vi "AlliGator Load Calibration Phasor Map.vi"(8 "Error In":errorcluster, 10 "File Path (empty: dialog)":path=path "", 11 "Calibration Phasor Map in":T1={"Phasor Frequency"=80000000.0, "Calibration Lifetime"=1e-09, "ROI Centers"=[], "ROI Descriptors"=[], "Map Resolution X"=0, "Map Resolution Y"=0, "z Array"=[]} {"ROI Descriptors"."Contours"."Type" items=["No Selection", "Point", "Line", "Rectangle", "Oval", "Polygon", "Freehand Region", "Annulus", "Unused2", "Unused3", "Broken Line", "Freehand Line", "Rotated Rectangle"]}) -> (0 "error out":errorcluster, 1 "Phasor Frequency":dbl[unit], 2 "File Path":path, 3 "Calibration Phasor Map out":T1={"Phasor Frequency"=80000000.0, "Calibration Lifetime"=1e-09, "ROI Centers"=[], "ROI Descriptors"=[], "Map Resolution X"=0, "Map Resolution Y"=0, "z Array"=[]} {"ROI Descriptors"."Contours"."Type" items=["No Selection", "Point", "Line", "Rectangle", "Oval", "Polygon", "Freehand Region", "Annulus", "Unused2", "Unused3", "Broken Line", "Freehand Line", "Rotated Rectangle"]}, 4 "Message":string)   [LabVIEW 2021, in "AlliGator Phasor Calibration.lvlib"]
doc: "Loads a <B>Phasor Calibraton Map</B>."
uses:
  AlliGator Phasor Calibration.lvlib
  Phasor/Phasor Calibration Map v2.ctl
  AlliGator Phasor Calibration Map v1.ctl
  c0370fcd-593d-4089-81d1-2cd858bd6d0b.vi
  f35317ec-b920-4f06-9f91-dc9fc3beab4a.vi
  f35317ec-b920-4f06-9f91-dc9fc3beab4a.vi/8a80743f-1319-44c8-96b0-3ef8fc688731.vi
  f35317ec-b920-4f06-9f91-dc9fc3beab4a.vi/931f4f8f-d8c6-4056-833f-5c8fe97b24b9.vi
  <vilib>/JDP Science/JSONtext/JSON text to Variant.vi
  <vilib>/Utility/error.llb/Error Cluster From Error Code.vi
  <vilib>/JDP Science/JSONtext/LVClass Serializer/JSONtext LVClass Serializer.lvclass
  <vilib>/ErrorRing/Error Ring.xnode
  Settings/AlliGator Settings.lvlib
  Time/Time.lvlib
  Phasor/Phasor.lvlib
panel:
  # "see the AlliGator License on the block diagram (Ctrl+E or Window:Show Block Diagram)"
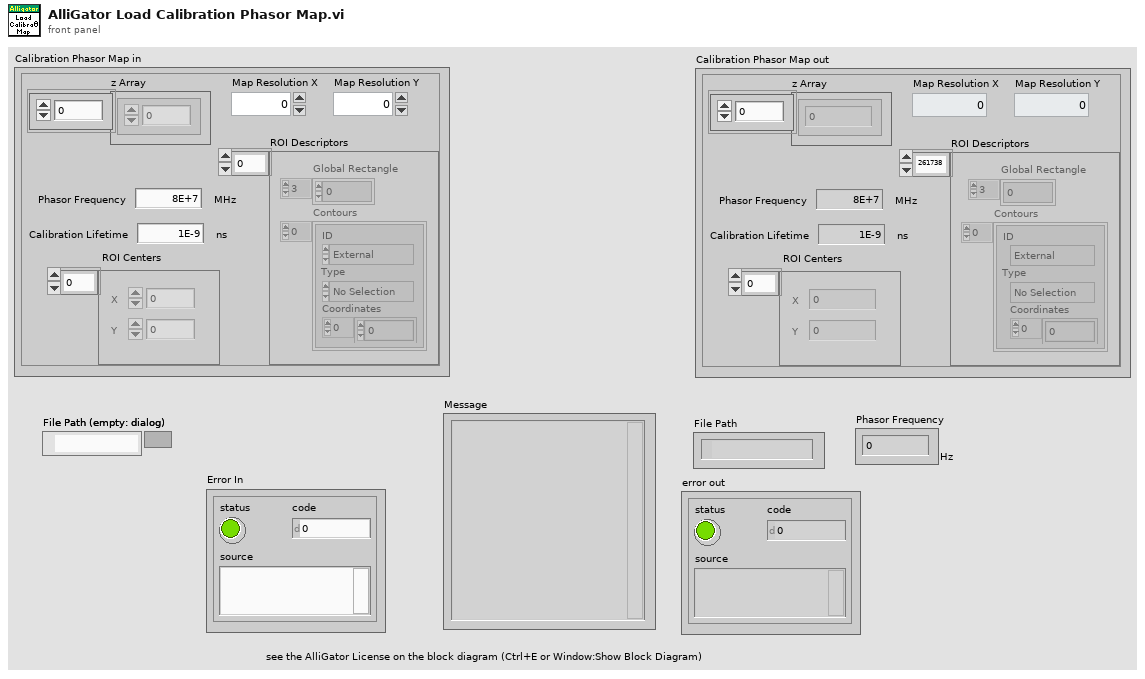
[diagram p1: front panel]
types:
  T1 = typedef "Phasor.lvlib/Phasor Calibration Map v2.ctl" = cluster{"Phasor Frequency":dbl[unit], "Calibration Lifetime":dbl[unit], "ROI Centers":cluster{"X":i32, "Y":i32}[], "ROI Descriptors":T2[], "Map Resolution X":i32, "Map Resolution Y":i32, "z Array":cdb[]}
  T2 = typedef "ROI Descriptor" = cluster{"Global Rectangle":i32[], "Contours":cluster{"ID":enum32{"External", "Internal"}, "Type":u32, "Coordinates":i32[]}[]}
  T3 = typedef "AlliGator Phasor Calibration.lvlib/AlliGator Phasor Calibration Map v1.ctl" = cluster{"m Array":dbl[], "phi Array":dbl[], "Phasor Frequency":dbl[unit], "Calibration Lifetime":dbl[unit], "ROI Centers":cluster{"X":i32, "Y":i32}[], "ROI Descriptors":T2[], "Map Resolution X":i32, "Map Resolution Y":i32}
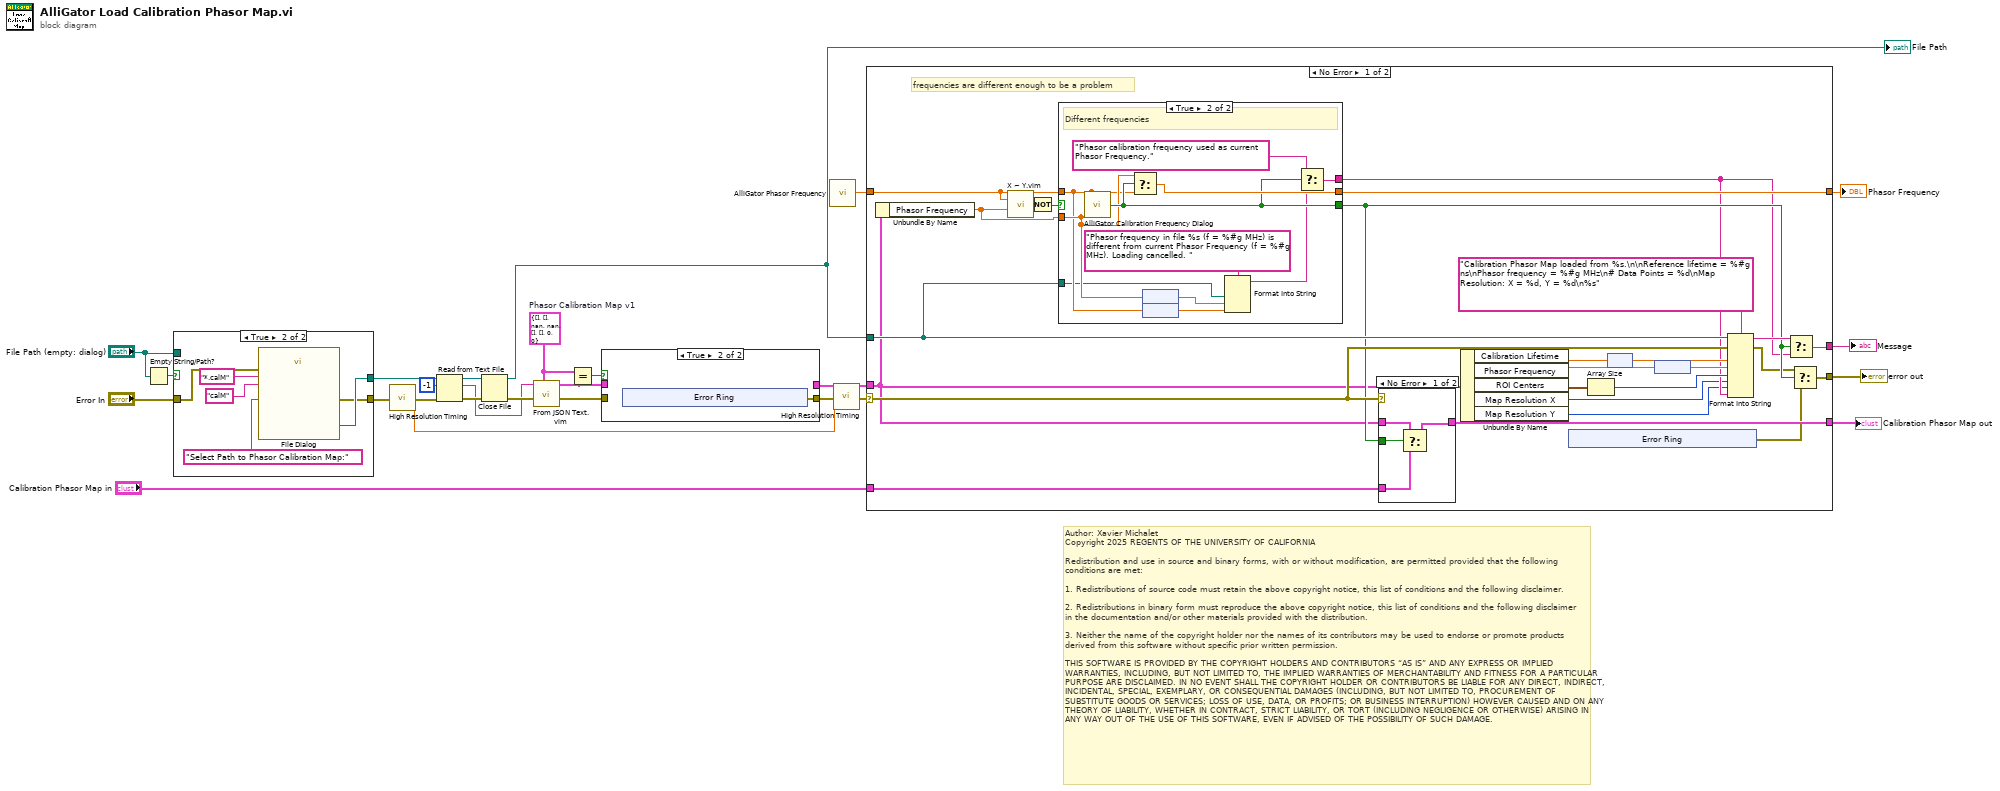
[diagram p0: block diagram]
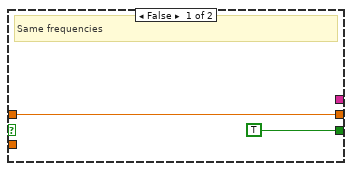
[diagram p3: hidden frame]
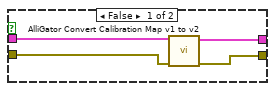
[diagram p5: hidden frame]
diagram:
  w14 = T3 {"m Array"=[], "phi Array"=[], "Phasor Frequency"=nan, "Calibration Lifetime"=nan, "ROI Centers"=[], "ROI Descriptors"=[], "Map Resolution X"=0, "Map Resolution Y"=0}  # Phasor Calibration Map v1
  # "Author: Xavier Michalet\nCopyright 2025 REGENTS OF THE UNIVERSITY OF CALIFORNIA\n\nRedistribution and use in source and binary forms, with or without modification, are permitted provided that the following conditions are met:\n\n1. Redistributions of source code must retain the above copyright notice, this list of conditions and the following disclaimer.\n\n2. Redistributions in binary form must reproduce the above copyright notice, this list of conditions and the following disclaimer in the documentation and/or other materials provided with the distribution.\n\n3. Neither the name of the copyright holder nor the names of its contributors may be used to endorse or promote products derived from this software without specific prior written permission.\n\nTHIS SOFTWARE IS PROVIDED BY THE COPYRIGHT HOLDERS AND CONTRIBUTORS “AS IS” AND ANY EXPRESS OR IMPLIED WARRANTIES, INCLUDING, BUT NOT LIMITED TO, THE IMPLIED WARRANTIES OF MERCHANTABILITY AND FITNESS FOR A PARTICULAR PURPOSE ARE DISCLAIMED. IN NO EVENT SHALL THE COPYRIGHT HOLDER OR CONTRIBUTORS BE LIABLE FOR ANY DIRECT, INDIRECT, INCIDENTAL, SPECIAL, EXEMPLARY, OR CONSEQUENTIAL DAMAGES (INCLUDING, BUT NOT LIMITED TO, PROCUREMENT OF SUBSTITUTE GOODS OR SERVICES; LOSS OF USE, DATA, OR PROFITS; OR BUSINESS INTERRUPTION) HOWEVER CAUSED AND ON ANY THEORY OF LIABILITY, WHETHER IN CONTRACT, STRICT LIABILITY, OR TORT (INCLUDING NEGLIGENCE OR OTHERWISE) ARISING IN ANY WAY OUT OF THE USE OF THIS SOFTWARE, EVEN IF ADVISED OF THE POSSIBILITY OF SUCH DAMAGE."
  n1 = Empty String/Path?(string/path="File Path (empty: dialog)") -> (empty?=w20:bool)
  n2 = case shown="True" w20 {
    tunnel: "Error In" -> [w27 w33]
    tunnel: [w28 w30] -> w22
    tunnel: [w27 w29] -> w21
    tunnel: "File Path (empty: dialog)" -> [w28 _]
    frame False {
    }
    frame True {
      n3 = call "File Dialog"("prompt"="Select Path to Phasor Calibration Map:" ("Prompt"), "error in"=w33, "pattern (all files)"="*.calM" ("pattern (*.xml)"), "pattern label"="calM" ("File Extension (xml)")) -> ("selected path"=w30:path, "error out"=w29:errorcluster)  [unwired: 8 in, 2 out]
    }
  }
  n4 = call "High Resolution Timing.vi"("Error In"=w21) -> ("elapsed (relative) seconds"=w17:dbl, "Error Out"=w18:errorcluster)  [unwired: 16 in, 1 out]
  n5 = Read from Text File(file (use dialog)=w22, count=-1, error in=w18) -> (refnum out=w24:refnum<file>, text=w15:string, error out=w25:errorcluster)  [unwired: 1 in, 1 out]
  n6 = Close File(refnum=w24, error in=w25) -> (path=w4:path, error out=w16:errorcluster)
  "File Path" <- w4
  n7 = call "From JSON Text.vim"("Data Type and Default Value"=w14, "error in (no error)"=w16, "JSON"=w15) -> ("error out"=w12:errorcluster, "Data out"=w11:T3)  [unwired: 7 in]
  n8 = Equal?(x=w14, y=w11) -> (x = y?=w10:bool)
  n9 = case shown="True" w10 {
    tunnel: w12 -> [w38 _]
    tunnel: [w37 w39] -> w13
    tunnel: [w36 _] -> w8
    tunnel: w11 -> [w35 _]
    frame False {
      n10 = call "AlliGator Convert Calibration Map v1 to v2.vi"("error in (no error)"=w38, "Phasor Calibration Map v1"=w35) -> ("error out"=w37:errorcluster, "Phasor Calibration Map v2"=w36:T1)  [unwired: 8 in]
    }
    frame True {
      n11 = xnode "Error Ring"() -> ("error out"=w39:errorcluster)
    }
  }
  n12 = call "AlliGator Phasor Frequency.vi"() -> ("Phasor Frequency"=w6:dbl[unit])
  n13 = call "High Resolution Timing.vi"("relative seconds (NaN)"=w17, "Error In"=w13) -> ("Error Out"=w9:errorcluster)  [unwired: 15 in, 2 out]
  n14 = case shown="No Error" w9 {
    selector: w9 -> [w62 w94]
    tunnel: [w68 w93] -> w5
    tunnel: "Calibration Phasor Map in" -> [w59 w93]
    tunnel: [w57 _] -> w3
    tunnel: w4 -> [w56 _]
    tunnel: [w55 w92] -> w1
    tunnel: [w52 w94] -> w2
    tunnel: w6 -> [w50 w92]
    tunnel: w8 -> [w49 _]
    frame No Error {
      # "frequencies are different enough to be a problem"
      n15 = Unbundle By Name(w49) -> ("Phasor Frequency"=w60:dbl[unit])
      n16 = call "X ~ Y.vim"("X"=w50, "Y"=w60) -> ("X ~= Y?"=w69:bool)  [unwired: 13 in]
      n17 = Not(x=w69) -> (.not. x?=w61:bool)
      n18 = case shown="True" w61 {
        tunnel: w50 -> [w80 w83]
        tunnel: w60 -> [_ w85]
        tunnel: [TRUE ("Use Calibration Frequency?") w89] -> w54
        tunnel: [w80 w91] -> w55
        tunnel: [_ w88] -> w46
        tunnel: w56 -> [_ w81]
        frame False {
          # "Same frequencies"
        }
        frame True {
          # "Different frequencies"
          n19 = call "AlliGator Calibration Frequency Dialog.vi"("Calibration Phasor Frequency"=w85, "Internal Phasor Frequency"=w83) -> ("Use Calibration Frequency?"=w89:bool)
          n20 = Select(t=w85, s=w89, f=w83) -> (s? t:f=w91:dbl[unit])
          n21 = node(w85) -> (w87:dbl)
          n22 = node(w83) -> (w84:dbl)
          n23 = Format Into String(format string="Phasor frequency in file %s (f = %#g MHz) is different from current Phasor Frequency (f = %#g MHz). Loading cancelled. ", w81, w87, w84) -> (resulting string=w82:string)  [unwired: 2 in, 1 out]
          n24 = Select(t="Phasor calibration frequency used as current Phasor Frequency." ("format string"), s=w89, f=w82) -> (s? t:f=w88:string)
        }
      }
      n25 = case shown="No Error" w62 {
        tunnel: w49 -> [w76 w78]
        tunnel: [w74 w78] -> w68
        tunnel: w59 -> [w75 _]
        tunnel: w54 -> [w77 _]
        frame No Error {
          n26 = Select(t=w76, s=w77, f=w75) -> (s? t:f=w74:T1)
        }
        frame Error {
        }
      }
      n27 = Unbundle By Name(w49) -> ("Calibration Lifetime"=w67:dbl[unit], "Phasor Frequency"=w66:dbl[unit], "ROI Centers"=w48:cluster{"X":i32, "Y":i32}[], "Map Resolution X"=w45:i32, "Map Resolution Y"=w44:i32)
      n28 = xnode "Error Ring"() -> ("error out"=w51:errorcluster)
      n29 = Array Size(array=w48) -> (size(s)=w47:i32)
      n30 = node(w67) -> (w65:dbl)
      n31 = node(w66) -> (w64:dbl)
      n32 = Format Into String(format string="Calibration Phasor Map loaded from %s.\n\nReference lifetime = %#g ns\nPhasor frequency = %#g MHz\n# Data Points = %d\nMap Resolution: X = %d, Y = %d\n%s", error in=w62, w56, w65, w64, w47, w45, w44, w46) -> (resulting string=w58:string, error out=w53:errorcluster)  [unwired: 1 in]
      n33 = Select(t=w58, s=w54, f=w46) -> (s? t:f=w57:string)
      n34 = Select(t=w53, s=w54, f=w51) -> (s? t:f=w52:errorcluster)
    }
    frame Error {
    }
  }
  "Calibration Phasor Map out" <- w5
  "error out" <- w2
  "Message" <- w3
  "Phasor Frequency" <- w1
